vi "1A Temperature Reader.vi"() -> ()   [LabVIEW 2011]
doc: "Elizabeth Mahon\n\nGets data from the cRIO's built-in temperature sensor and sends it up to the computer. Talks to the FPGA, sends it out through a FIFO."
uses:
  <vilib>/rvi/eio/common/nirviEmuTemplateMethod_errors.vi
  <vilib>/rvi/DataTransferAndStorage/Container/Common/niFpgaContainerExecOnDevCompGetState.vi
  <vilib>/rvi/FIFO/Fifo_Resource/nirvififoEmulationSetSize.vi
  <vilib>/rvi/DataTransferAndStorage/Container/Common/niFpgaContainerGetUniqueNameForEmu.vi
  <vilib>/rvi/interface/RandomDataEmulation/nirviRandomDataFPGAFIFO.vi
  <vilib>/rvi/interface/RandomDataEmulation/niFpgaRandomDataHandleErrors.vi
  <vilib>/rvi/eio/common/nirviEmuReportErrorAndStop.vi
  <vilib>/eio/EIONode/EIONode.xnode
  <vilib>/rvi/DataTransferAndStorage/Container/XNode/niFpgaContainer.xnode
  <vilib>/rvi/FIFO/Fifo_Resource/niFpgaFifoEmulationRefIn.vi
panel:
  in  "stop":bool
  out "Temperature":i16(graph)
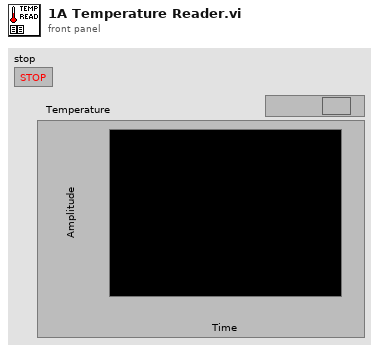
[diagram p1: front panel]
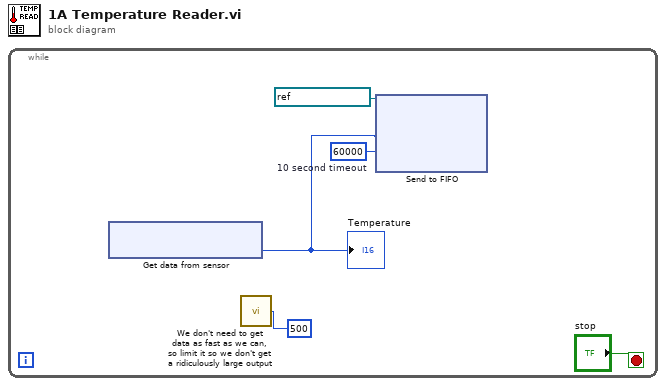
[diagram p0: block diagram]
diagram:
  n1 = while {
    stop <- "stop" stop-if-true
    w3 = 60000  # 10 second timeout
    n2 = xnode "Get data from sensor"() -> ("Chassis Temperature"=w4:i16)  [unwired: 1 in, 1 out]
    "Temperature" <- w4
    n3 = call "We don't need to get data as fast as we can, so limit it so we don't get a ridiculously large output"("Count(mSec)"=u32 500) -> ()  [unwired: 1 out]
    n4 = xnode "Send to FIFO"("Element"=w4, "Timeout"=w3, "FIFO In"=refnum<k21> "Temperature") -> ()  [unwired: 2 out]
  }
